vi "Analog_enable.vi"(8 "error in":errorcluster) -> (0 "error out":errorcluster)   [LabVIEW 2018]
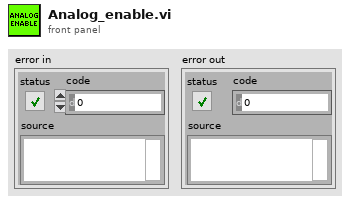
[diagram p1: front panel]
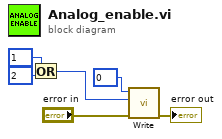
[diagram p0: block diagram]
diagram:
  n1 = Or(x=u8 1 ("Slave Address (7-bit)"), y=u8 2 ("Slave Address (7-bit)")) -> (x .or. y?=w1:u8)
  n2 = call "Write.vi"("error in"="error in", "Data to write"=w1, "Address"=u8 0 ("Slave Address (7-bit)")) -> ("error out"=→"error out":errorcluster)  [unwired: 8 in]
